vi "Step Association Get By Station and Step.vi"(8 "error in (no error)":errorcluster, 9 "iStep (0)":i32, 10 "iStation (0)":i32, 11 "Connection Refnum":T2) -> (0 "error out":errorcluster, 2 "Step Associations":T1[](array[typedef]), 3 "Connection Refnum":T2, 4 "Data Present?":bool)   [LabVIEW 2011]
uses:
  Summitek EXT/ODBC/SQL Controls/Connection Refnum.ctl
  Step Association Record.ctl
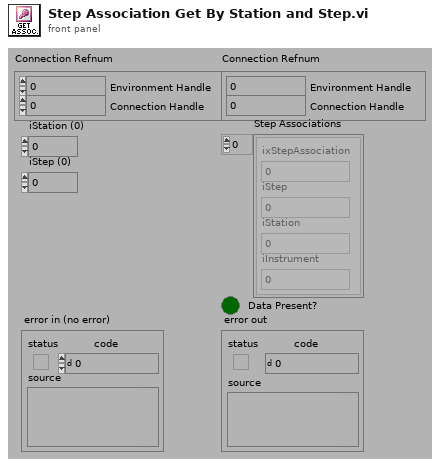
[diagram p1: front panel]
types:
  T1 = typedef "Step Association Record.ctl" = cluster{"ixStepAssociation":i32, "iStep":i32, "iStation":i32, "iInstrument":i32}
  T2 = typedef "Connection Refnum.ctl" = cluster{"Environment Handle":i32, "Connection Handle":i32}
  T3 = typedef "Statement Refnum.ctl" = cluster{"Statement Handle":i32, "Parameter Number":u16}
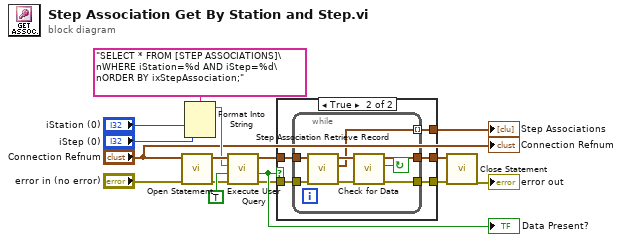
[diagram p0: block diagram]
diagram:
  n1 = call "Open Statement.vi"("error in (no error)"="error in (no error)", "Connection Refnum"="Connection Refnum") -> ("error out"=w8:errorcluster, "Statement Refnum"=w9:T3)  [unwired: 4 out]
  n2 = Format Into String(format string="SELECT * FROM [STEP ASSOCIATIONS]\nWHERE iStation=%d AND iStep=%d\nORDER BY ixStepAssociation;" ("User Query"), "iStation (0)", "iStep (0)") -> (resulting string=w7:string)  [unwired: 2 in, 1 out]
  n3 = call "Execute User Query.vi"("error in (no error)"=w8, "Return Data? (f)"=TRUE, "User Query"=w7, "Statement Refnum"=w9) -> ("error out"=w15:errorcluster, "Data Present?"=w16:bool, "Statement Refnum"=w14:T3)  [unwired: 1 out]
  "Data Present?" <- w16
  n4 = case shown="True" w16 {
    tunnel: w15 -> [w17 w23]
    tunnel: w14 -> [w18 w22]
    tunnel: [w17 w21] -> w11
    tunnel: [w18 w20] -> w12
    tunnel: [_ w19] -> w4
    frame False {
    }
    frame True {
      n5 = while {
        tunnel: w23 -> [w31]
        tunnel: w22 -> [w30]
        tunnel: [w24] -> w19 mode=indexing
        tunnel: [w27] -> w21
        tunnel: [w26] -> w20
        stop <- w25 continue-if-true
        n6 = call "Step Association Retrieve Record.vi"("error in (no error)"=w31, "Statement Refnum"=w30) -> ("error out"=w28:errorcluster, "Association"=w24:T1, "Statement Refnum"=w29:T3)  [unwired: 7 in]
        n7 = call "Check for Data.vi"("error in (no error)"=w28, "Statement Refnum"=w29) -> ("error out"=w27:errorcluster, "Data Present?"=w25:bool, "Statement Refnum"=w26:T3)  [unwired: 3 out]
      }
    }
  }
  "Step Associations" <- w4
  n8 = call "Close Statement.vi"("error in (no error)"=w11, "Statement Refnum"=w12) -> ("error out"=→"error out":errorcluster)  [unwired: 5 out]
  "Connection Refnum" <- "Connection Refnum"
